vi "Polynomial GCD Pair (CDB).vi"(9 "tolerance":dbl=1e-08, 10 "Q(x)":cdb[](array[numeric]), 11 "P(x)":cdb[](array[numeric])) -> (0 "error":i32, 1 "Co-factor of Q(x)":cdb[](array[numeric]), 2 "Co-factor of P(x)":cdb[](array[numeric]), 3 "Greatest Common Divisor":cdb[](array[numeric]))   [LabVIEW 2020, in "NI_AALPro.lvlib"]
uses:
  NI_AALPro.lvlib
  <resource>/lvanlys.dll
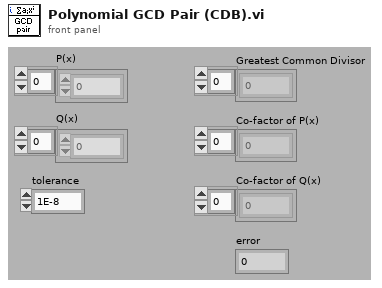
[diagram p1: front panel]
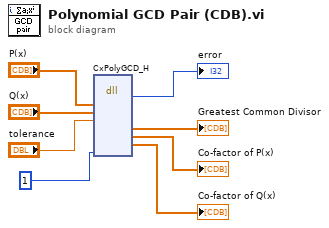
[diagram p0: block diagram]
diagram:
  n1 = dll-call lib="C:/Program Files (x86)/National Instruments/LabVIEW 2020/resource/lvanlys.*" fn="CxPolyGCD_H"("P(x)"="P(x)", "Q(x)"="Q(x)", "tol"="tolerance", "isLCM"=1) -> (→"error":i32, "Greatest Common Divisor"=→"Greatest Common Divisor":cdb[], "Co-factor of P(x)"=→"Co-factor of P(x)":cdb[], "Co-factor of Q(x)"=→"Co-factor of Q(x)":cdb[])  [unwired: 10 in, 2 out]
